vi "Intake Immediate.vi"(7 "Description":string, 8 "Command Info In":T1, 9 "Deadband Value":dbl=0.01, 10 "IntakeLift":dbl, 11 "WheelSpeed":dbl) -> (0 "Command Info Out":T1)   [LabVIEW 2019]
doc: "This template includes code for deadband comparision to avoid excessive command scheduling. It is particularly useful for joystick-driven commands.\n\nBe sure to right-click and select New from Template and save with a new command name."
uses:
  <vilib>/Rock Robotics/WPI/Framework/Command Status Info.ctl
  <vilib>/Rock Robotics/WPI/Framework/Completion Status.ctl
  <vilib>/Rock Robotics/WPI/Framework/Completion Notifier.ctl
  Implementation/Intake Setpoints.ctl
  Implementation/Intake Operations.ctl
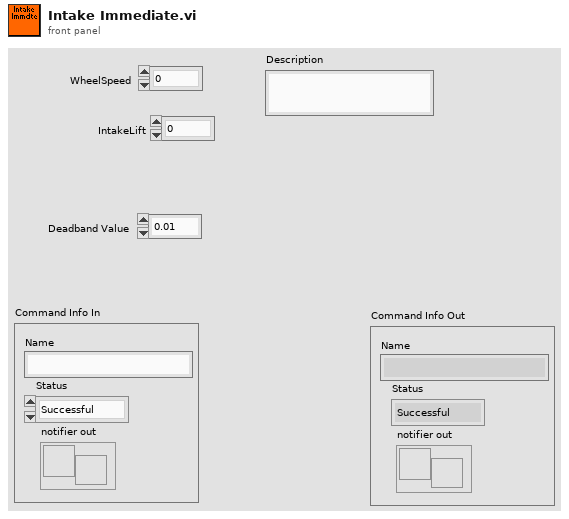
[diagram p1: front panel]
types:
  T1 = typedef "Command Status Info.ctl" = cluster{"Name":string, "Status":T2, "notifier out":T3}
  T2 = typedef "Completion Status.ctl" = enum16{"Successful", "Aborted", "Incomplete"}
  T3 = typedef "Completion Notifier.ctl" = refnum<notifier>
  T4 = typedef "Intake Setpoints.ctl" = cluster{"Operation":T5, "Setpoint":dbl, "Duration":dbl, "Flip Analog":dbl}
  T5 = typedef "Intake Operations.ctl" = enum16{"Reserve", "Read Current", "Intake until Full", "Immediate", "Flip on Push", "Intake for time"}
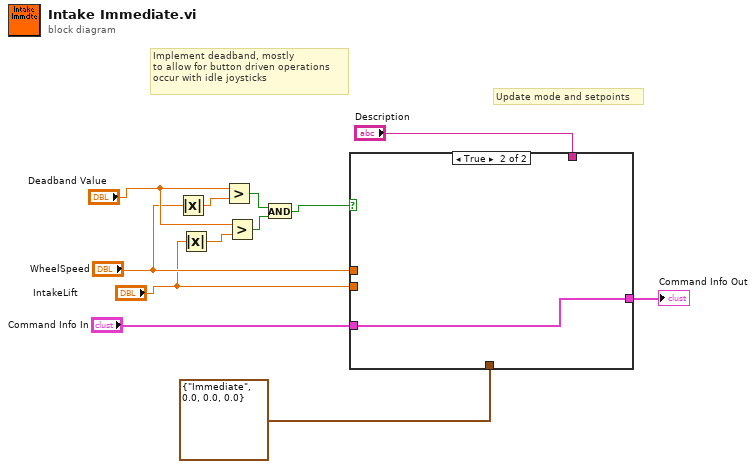
[diagram p0: block diagram]
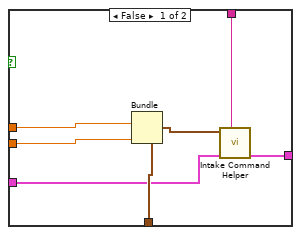
[diagram p2: hidden frame]
diagram:
  # "Implement deadband, mostly\nto allow for button driven operations\noccur with idle joysticks"
  # "Update mode and setpoints"
  n1 = Absolute Value(x="WheelSpeed") -> (abs(x)=w8:dbl)
  n2 = Absolute Value(x="IntakeLift") -> (abs(x)=w6:dbl)
  n3 = Greater?(x="Deadband Value", y=w8) -> (0:w7:bool)
  n4 = Greater?(x="Deadband Value", y=w6) -> (0:w5:bool)
  n5 = And(x=w7, y=w5) -> (x .and. y?=w1:bool)
  n6 = case shown="True" w1 {
    tunnel: "WheelSpeed" -> [w19 _]
    tunnel: T4 {"Operation"=enum."Immediate", "Setpoint"=0.0, "Duration"=0.0, "Flip Analog"=0.0} ("SubSystem Data") -> [w18 _]
    tunnel: [w17 w20] -> w12
    tunnel: "Command Info In" -> [w16 w20]
    tunnel: "Description" -> [w15 _]
    tunnel: "IntakeLift" -> [w14 _]
    frame False {
      n7 = Bundle(cluster=w18, "Setpoint"=w19, "Flip Analog"=w14) -> (w13:T4)  [unwired: 2 in]
      n8 = call "Intake Command Helper.vi"("Description"=w15, "Command Info In"=w16, "SubSystem Data"=w13) -> ("Command Info Out"=w17:T1)  [unwired: 6 in, 2 out]
    }
    frame True {
    }
  }
  "Command Info Out" <- w12
